vi "Send Aircraft Message.vi"(8 "error in (no error)":errorcluster, 10 "Aircraft ID":u8, 11 "MAVLink Message":u8[](array[numeric])) -> (0 "error out":errorcluster)   [LabVIEW 2014]
uses:
  Ground Station to Aircraft Coms/SubVI/Aircraft Data Router/SubVI/Queue References/SubVI/Get Aircraft TX Queue String.vi
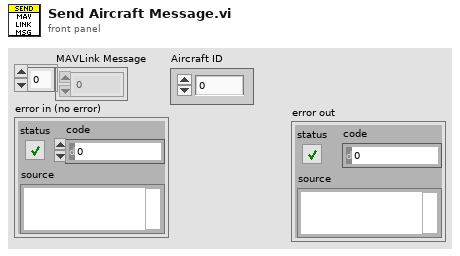
[diagram p1: front panel]
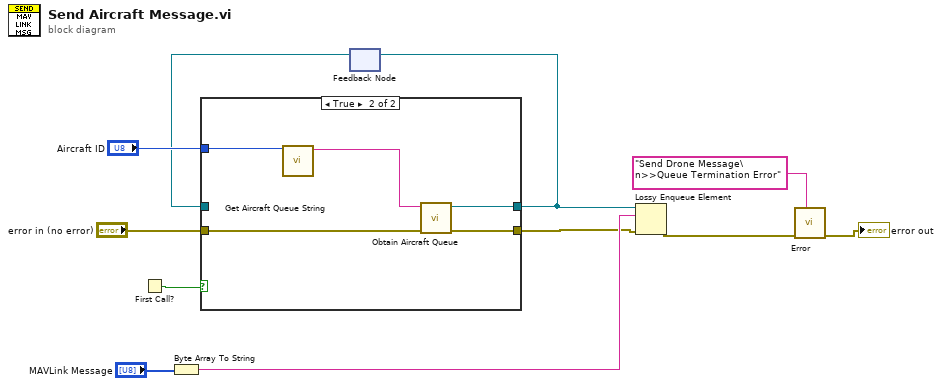
[diagram p0: block diagram]
diagram:
  n1 = First Call?() -> (First Call?: T/F=w6:bool)
  n2 = Byte Array To String(unsigned byte array="MAVLink Message") -> (string=w10:string)
  n3 = feedback #1() -> (w4:refnum<queue>)  [unwired: 1 in]
  n4 = case shown="True" w6 {
    tunnel: "Aircraft ID" -> [_ w18]
    tunnel: [w13 w17] -> w5
    tunnel: [w12 w16] -> w8
    tunnel: "error in (no error)" -> [w12 w14]
    tunnel: w4 -> [w13 _]
    frame False {
    }
    frame True {
      n5 = call-poly "Get Aircraft Queue String.vi"("Aircraft ID"=w18) -> ("Aircraft Queue Name"=w15:string)  [unwired: 9 in, 1 out]
      n6 = call "Obtain Aircraft Queue.vi"("error in (no error)"=w14, "Queue Name"=w15) -> ("error out"=w16:errorcluster, "queue out"=w17:refnum<queue>)  [unwired: 8 in]
    }
  }
  n7 = feedback-in #1(w5) -> ()
  n8 = Lossy Enqueue Element(queue=w5, element=w10, error in (no error)=w8) -> (error out=w2:errorcluster)  [unwired: 3 out]
  n9 = call "Error.vi"("Error Message"="Send Drone Message\n>>Queue Termination Error", "Error In"=w2) -> ("Error Out"=→"error out":errorcluster)  [unwired: 9 in]
